vi "FeedBack Chanel.vi"(0 "Test Name":string, 1 "Lvdt":refnum<vi>, 5 "Channels (Int)":i32[](array[numeric]), 7 "FeedBack Channel":string[](array[string])=["fgdgfvcbc", "vnfhgjkn", "21354682"], 9 "Wait/Poll (ms)":u32, 11 "Parameter":u8) -> (4 "Out":i32, 6 "Array":bool[](array[boolean]), 10 "Fail":bool, 12 "Input Status":bool[](array[boolean]), 13 "Channel No":i32[](array[numeric]))   [LabVIEW 2020]
uses:
  Galobal variable_TI.vi
  Project Setup/Globle Variable/GR_Servo.vi
panel:
  out "Pokayoka Result":cluster{"Sensor Name":string, "Boolean":bool}[](array[cluster])
  out "output array":bool[](array[boolean])
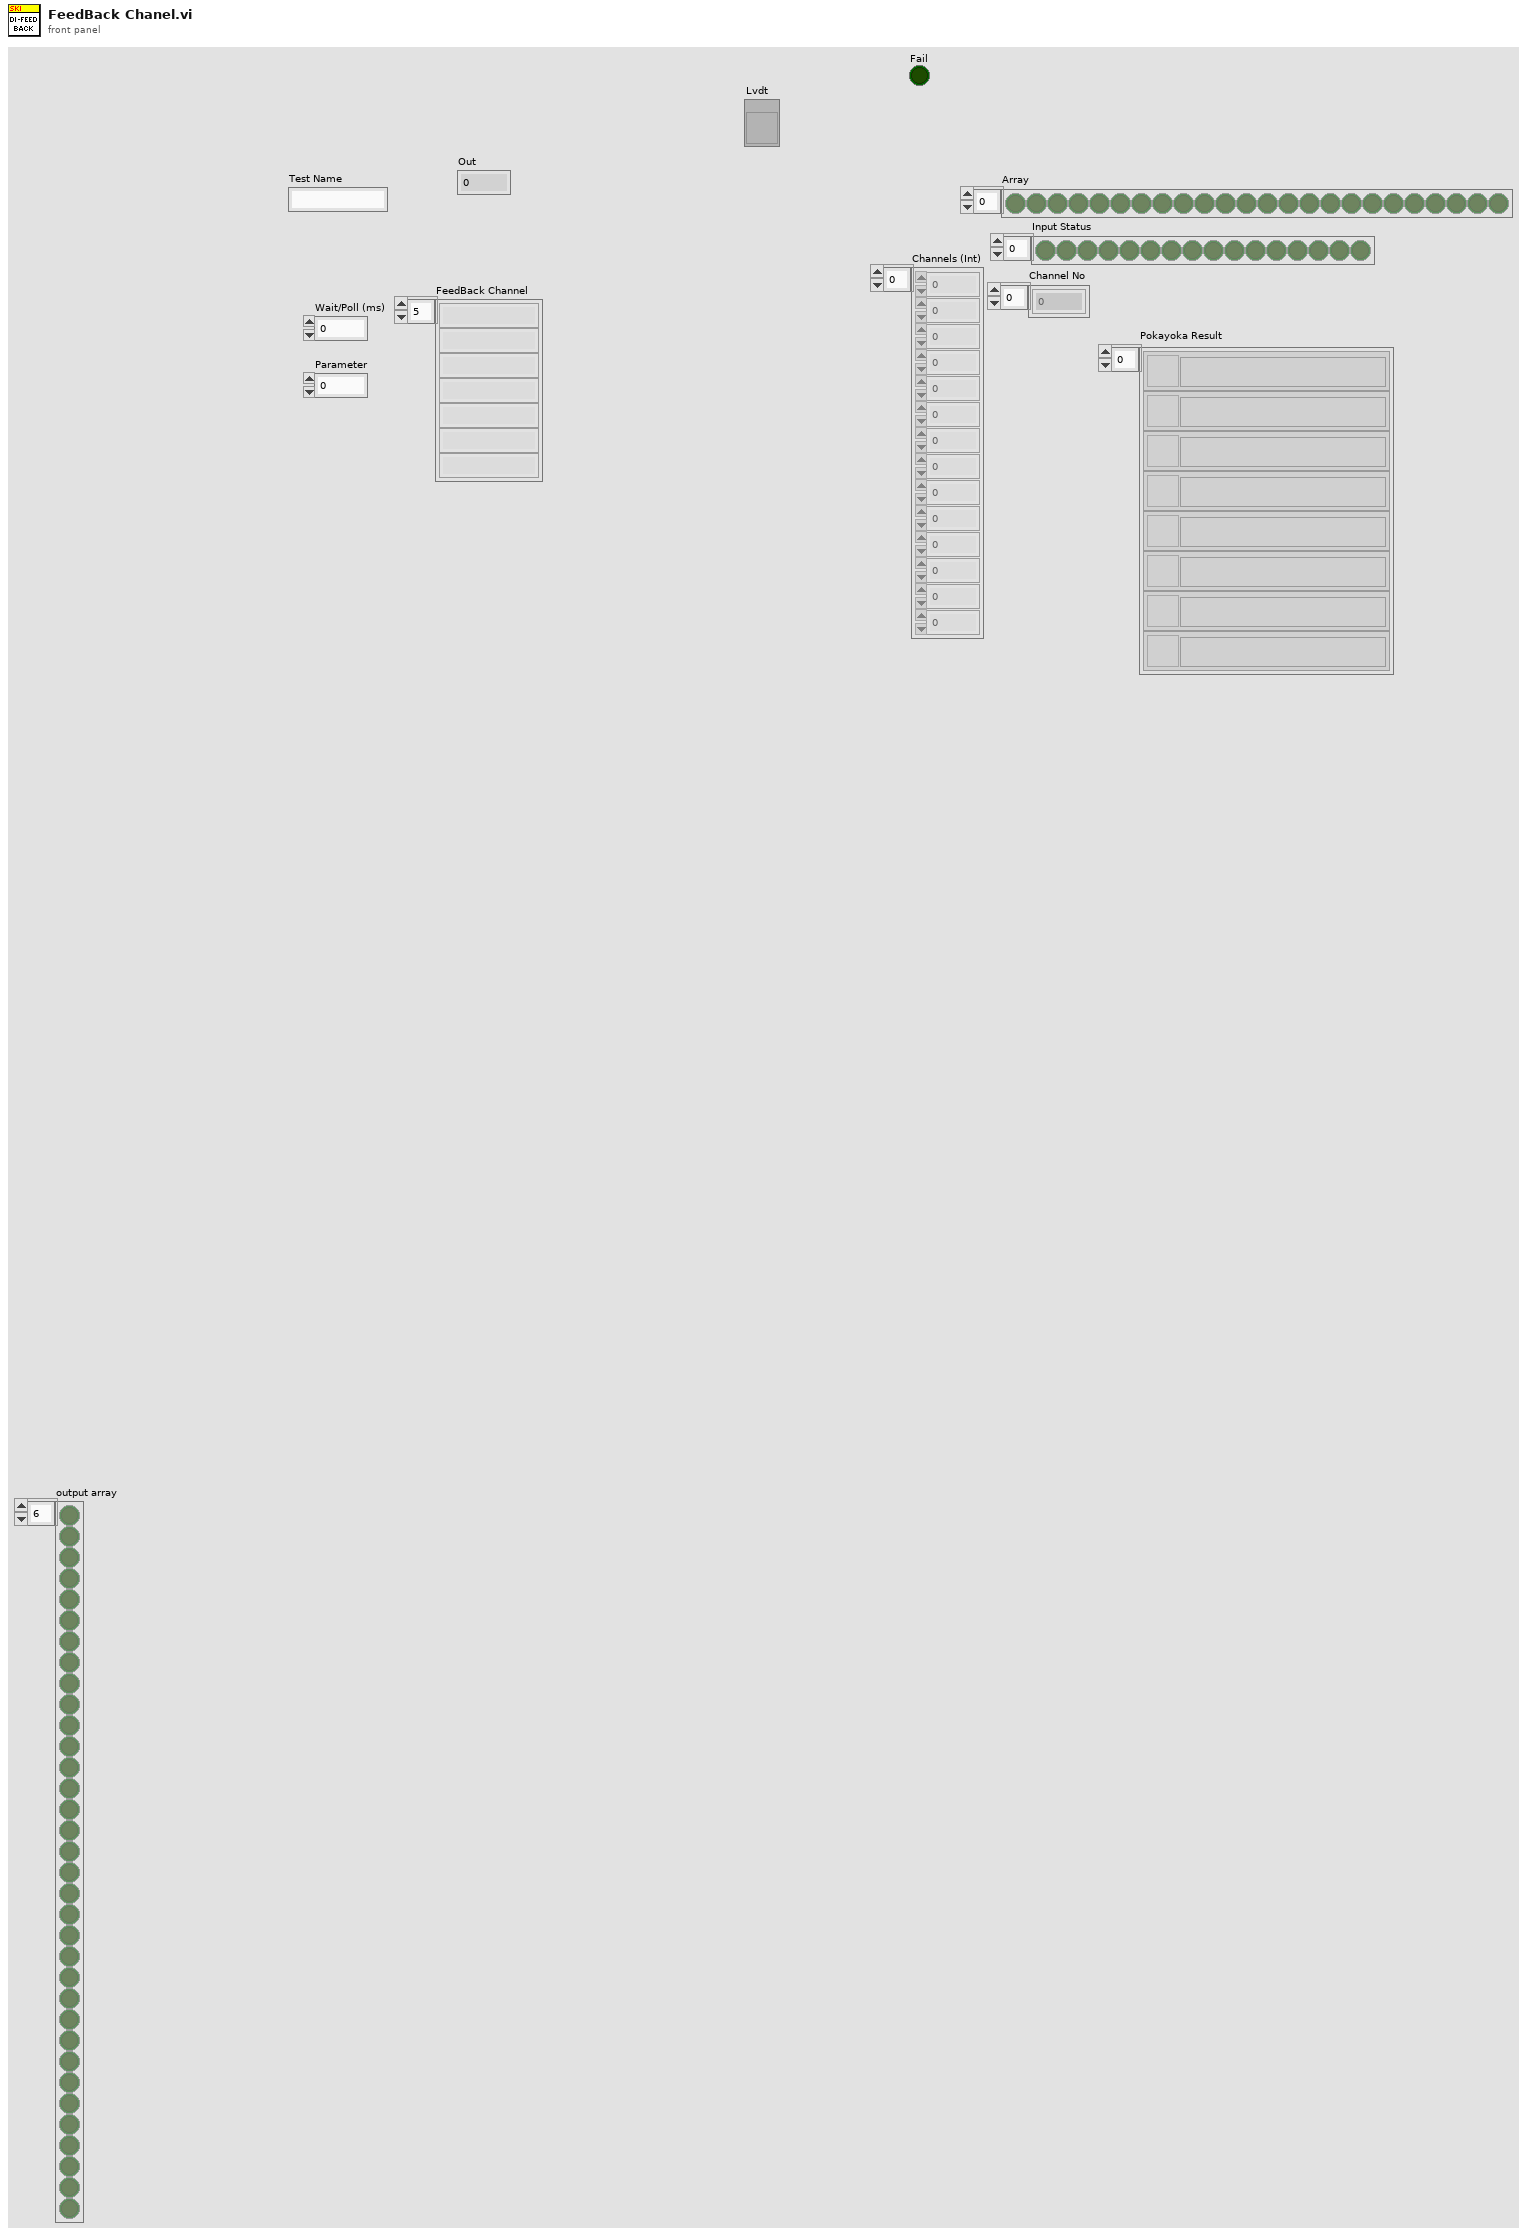
[diagram p1: front panel]
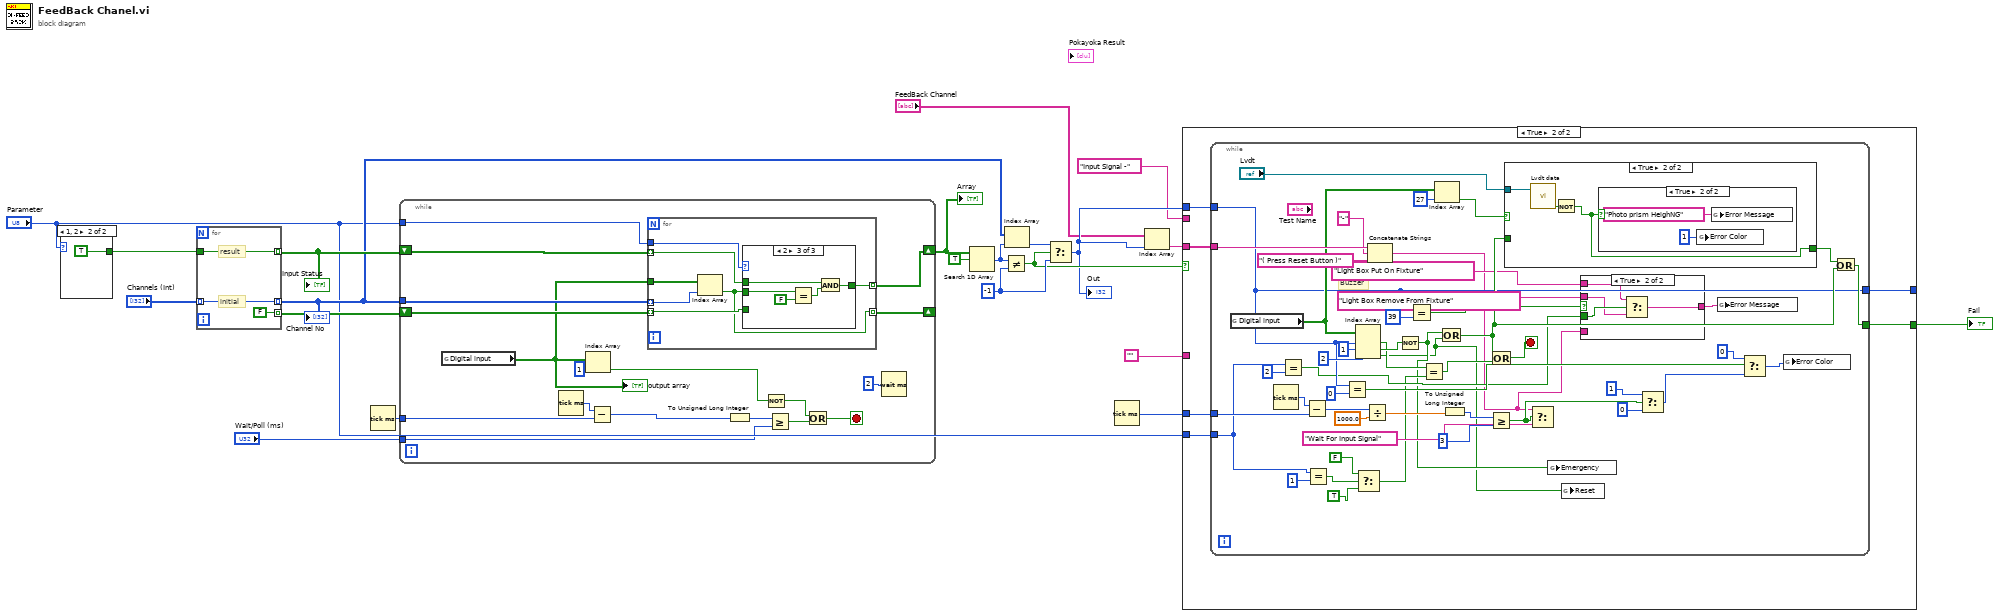
[diagram p0: block diagram]
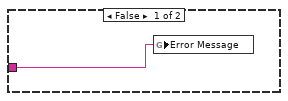
[diagram p2: hidden frame]
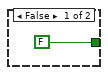
[diagram p4: hidden frame]
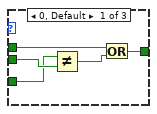
[diagram p6: hidden frame]
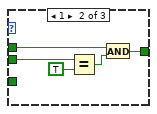
[diagram p7: hidden frame]
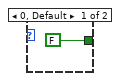
[diagram p8: hidden frame]
diagram:
  w21 = -1 ("y")
  n1 = case shown="1, 2" "Parameter" {
    tunnel: [FALSE TRUE] -> w12
    frame 0, Default {
    }
    frame 1, 2 {
    }
  }
  n2 = for {
    tunnel: [w26] -> w7 mode=indexing
    tunnel: w12 -> [w26]
    tunnel: "Channels (Int)" -> [w25] mode=indexing
    tunnel: [w25] -> w6 mode=indexing
    tunnel: [FALSE] -> w16 mode=indexing
    # "result"
    # "initial"
  }
  "Input Status" <- w7
  "Channel No" <- w6
  n3 = Tick Count (ms)() -> (millisecond timer value=w15:u32)
  n4 = while {
    tunnel: "Wait/Poll (ms)" -> [w32]
    tunnel: w15 -> [w43]
    tunnel: w6 -> [w41]
    tunnel: "Parameter" -> [w40]
    shift-right: [w39] -> w18
    shift-left: w7 -> [w37]
    shift-right: [w38] -> _
    shift-left: w16 -> [w36]
    stop <- w34 stop-if-true
    n5 = global read "Galobal variable_TI.vi" "Digital input"() -> (w28:bool[])
    "output array" <- w28
    n6 = Tick Count (ms)() -> (millisecond timer value=w44:u32)
    n7 = Index Array(array=w28, index=1) -> (element=w30:bool)
    n8 = Subtract(x=w44, y=w43) -> (x-y=w27:u32)
    n9 = for {
      tunnel: w36 -> [w46] mode=indexing
      tunnel: w37 -> [w48] mode=indexing
      tunnel: w28 -> [w51]
      tunnel: w41 -> [w50] mode=indexing
      tunnel: w40 -> [w49]
      tunnel: [w47] -> w39 mode=indexing
      tunnel: [w45] -> w38 mode=indexing
      n10 = Index Array(array=w51, index=w50) -> (element=w45:bool)
      n11 = case shown="2" w49 {
        tunnel: w45 -> [w56 w59 w66]
        tunnel: w48 -> [w54 w58 w63]
        tunnel: [w52 w57 w62] -> w47
        tunnel: w46 -> [w55 _ _]
        frame 0, Default {
          n12 = Not Equal?(x=w55, y=w56) -> (x != y?=w53:bool)
          n13 = Or(x=w54, y=w53) -> (x .or. y?=w52:bool)
        }
        frame 1 {
          n14 = Equal?(x=w59, y=TRUE) -> (x = y?=w60:bool)
          n15 = And(x=w58, y=w60) -> (x .and. y?=w57:bool)
        }
        frame 2 {
          n16 = Equal?(x=w66, y=FALSE) -> (x = y?=w64:bool)
          n17 = And(x=w63, y=w64) -> (x .and. y?=w62:bool)
        }
      }
    }
    n18 = To Unsigned Long Integer(number=w27) -> (unsigned 32bit integer=w42:u32)
    n19 = Not(x=w30) -> (.not. x?=w31:bool)
    n20 = Greater Or Equal?(x=w42, y=w32) -> (x >= y?=w35:bool)
    n21 = Or(x=w31, y=w35) -> (x .or. y?=w34:bool)
    n22 = Wait (ms)(milliseconds to wait=u32 2) -> ()  [unwired: 1 out]
  }
  "Array" <- w18
  n23 = Search 1D Array(1D array=w18, element=TRUE) -> (index of element=w19:i32)  [unwired: 1 in]
  n24 = Not Equal?(x=w19, y=w21) -> (x != y?=w11:bool)
  n25 = Index Array(array=w6, index=w19) -> (element=w20:i32)
  n26 = Select(t=w20, s=w11, f=w21) -> (s? t:f=w10:i32)
  "Out" <- w10
  n27 = Tick Count (ms)() -> (millisecond timer value=w4:u32)
  n28 = Index Array(array="FeedBack Channel", index=w10) -> (element=w9:string)
  n29 = case shown="True" w11 {
    tunnel: w10 -> [_ w72]
    tunnel: w9 -> [_ w73]
    tunnel: "Input Signal -" ("string") -> [_ _]
    tunnel: w4 -> [_ w71]
    tunnel: "" -> [w67 _]
    tunnel: [_ w70] -> _
    tunnel: "Parameter" -> [_ w69]
    tunnel: [_ w68] -> w1
    frame False {
      n30 = global write "GR_Servo.vi" "Error Message"(w67) -> ()
    }
    frame True {
      n31 = while {
        tunnel: w73 -> [w122]
        tunnel: w72 -> [w91]
        tunnel: w71 -> [w117]
        tunnel: [w91] -> w70
        tunnel: w69 -> [w83]
        tunnel: [w99] -> w68
        stop <- w108 stop-if-true
        # "Buzzer"
        n32 = global read "Galobal variable_TI.vi" "Digital input"() -> (w107:bool[])
        n33 = Tick Count (ms)() -> (millisecond timer value=w120:u32)
        n34 = Equal?(x=w83, y=u8 2) -> (x = y?=w85:bool)
        n35 = Subtract(x=w120, y=w117) -> (x-y=w119:u32)
        n36 = Equal?(x=w83, y=u8 1) -> (x = y?=w82:bool)
        n37 = Equal?(x=w91, y=0) -> (x = y?=w97:bool)
        n38 = Index Array(array=w107, index #1=w91, index #2=1 ("index"), index #3=2 ("index")) -> (element #1=w79:bool, element #2=w110:bool, element #3=w75:bool)
        n39 = Select(t=FALSE, s=w82, f=TRUE) -> (s? t:f=w77:bool)
        n40 = Divide(x=w119, y=1000.0) -> (x/y=w114:dbl)
        n41 = Concatenate Strings(w122, "-" ("string"), "( Press Reset Button )" ("string")) -> (w74:string)
        n42 = Not(x=w110) -> (.not. x?=w76:bool)
        n43 = Equal?(x=w91, y=39) -> (x = y?=w89:bool)
        n44 = Equal?(x=w79, y=w77) -> (x = y?=w78:bool)
        n45 = Index Array(array=w107, index=27) -> (element=w105:bool)
        n46 = Compound Arithmetic op=OR(w76, w75) -> (w100:bool)
        n47 = To Unsigned Long Integer(number=w114) -> (unsigned 32bit integer=w116:u32)
        n48 = Greater Or Equal?(x=w116, y=u32 3) -> (x >= y?=w103:bool)
        n49 = Compound Arithmetic op=OR(w100, w78) -> (w108:bool)
        n50 = case shown="True" w105 {
          tunnel: "Lvdt" -> [_ w131]
          tunnel: [FALSE w129] -> w101
          tunnel: w100 -> [_ _]
          frame False {
          }
          frame True {
            n51 = call "Lvdt data.vi"("Lvdt"=w131) -> ("LVDT"=w130:bool)  [unwired: 8 in, 2 out]
            n52 = Not(x=w130) -> (.not. x?=w129:bool)
            n53 = case shown="True" w129 {
              frame False {
              }
              frame True {
                n54 = global write "GR_Servo.vi" "Error Color"(1 ("Error Color")) -> ()
                n55 = global write "GR_Servo.vi" "Error Message"("Photo prism HeighNG" ("Error Message")) -> ()
              }
            }
          }
        }
        n56 = Select(t=w74, s=w103, f="Wait For Input Signal") -> ()  [unwired: 1 out]
        n57 = global write "Galobal variable_TI.vi" "Emergency"(w76) -> ()
        n58 = global write "Galobal variable_TI.vi" "Reset"(w75) -> ()
        n59 = case shown="True" w89 {
          tunnel: w85 -> [_ w127]
          tunnel: "LIght Box Put On Fixture" ("f") -> [_ w126]
          tunnel: "Light Box Remove From Fixture" ("f") -> [_ w125]
          tunnel: [w123 w124] -> w86
          tunnel: w74 -> [w123 _]
          frame False {
          }
          frame True {
            n60 = Select(t=w126, s=w127, f=w125) -> (s? t:f=w124:string)
          }
        }
        n61 = Select(t=1 ("y"), s=w103, f=0) -> (s? t:f=w94:i32)
        n62 = global write "GR_Servo.vi" "Error Message"(w86) -> ()
        n63 = Select(t=0 ("y"), s=w97, f=w94) -> (s? t:f=w93:i32)
        n64 = global write "GR_Servo.vi" "Error Color"(w93) -> ()
        n65 = Or(x=w101, y=w100) -> (x .or. y?=w99:bool)
      }
    }
  }
  "Fail" <- w1
